vi "rhythm game.vi"() -> ()   [LabVIEW 2023]
uses:
  <vilib>/numeric/Random Number (Range) DBL.vi
  be73d2ca-6044-4015-8fdc-046309639c3a.vi
  e82d1244-044b-4f16-bbdc-f3884a827bcd.vi
  <vilib>/Utility/inputDevices.llb/keyboardAcquire.vi
panel:
  out "fg":picture
  in  "stop":bool
  out "bg":picture
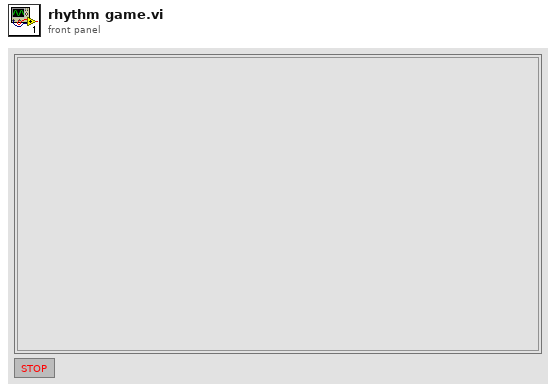
[diagram p1: front panel]
types:
  T1 = cluster{"1st rail":cluster{"key":enum16{"0", "1", "2", "3", "4", "5", "6", "7", "8", "9", "A", "B", "C", "D", "E", "F", "G", "H", "I", "J", "K", "L", "M", "N", "O", "P", "Q", "R", "S", "T", "U", "V", "W", "X", "Y", "Z", "F1", "F2", "F3", "F4", "F5", "F6", "F7", "F8", "F9", "F10", "F11", "F12", "F13", "F14", "F15", "ADD", "BACK", "BACKSLASH", "CAPITAL", "COMMA", "DECIMAL", "DELETE", "DIVIDE", "DOWN", "END", "EQUALS", "ESCAPE", "GRAVE (`)", "HOME", "INSERT", "LBRACKET", "LCONTROL", "LEFT", "L ALT", "LSHIFT", "LWIN", "MINUS", "MULTIPLY", "NEXT", "NUMLOCK", "NUMPAD_0", "NUMPAD_1", "NUMPAD_2", "NUMPAD_3", "NUMPAD_4", "NUMPAD_5", "NUMPAD_6", "NUMPAD_7", "NUMPAD_8", "NUMPAD_9", "PAUSE", "PERIOD", "PRIOR (PG UP)", "RBRACKET", "RCONTROL", "RETURN", "RIGHT", "R ALT", "RSHIFT", "RWIN", "SCROLL", "SEMICOLON", "SLASH", "SPACE", "SUBTRACT", "TAB", "UP", "ENTER (num pad)", "' (quote)"}, "note index":i32, "note acc":i32}, "2nd rail":cluster{"key":enum16{"0", "1", "2", "3", "4", "5", "6", "7", "8", "9", "A", "B", "C", "D", "E", "F", "G", "H", "I", "J", "K", "L", "M", "N", "O", "P", "Q", "R", "S", "T", "U", "V", "W", "X", "Y", "Z", "F1", "F2", "F3", "F4", "F5", "F6", "F7", "F8", "F9", "F10", "F11", "F12", "F13", "F14", "F15", "ADD", "BACK", "BACKSLASH", "CAPITAL", "COMMA", "DECIMAL", "DELETE", "DIVIDE", "DOWN", "END", "EQUALS", "ESCAPE", "GRAVE (`)", "HOME", "INSERT", "LBRACKET", "LCONTROL", "LEFT", "L ALT", "LSHIFT", "LWIN", "MINUS", "MULTIPLY", "NEXT", "NUMLOCK", "NUMPAD_0", "NUMPAD_1", "NUMPAD_2", "NUMPAD_3", "NUMPAD_4", "NUMPAD_5", "NUMPAD_6", "NUMPAD_7", "NUMPAD_8", "NUMPAD_9", "PAUSE", "PERIOD", "PRIOR (PG UP)", "RBRACKET", "RCONTROL", "RETURN", "RIGHT", "R ALT", "RSHIFT", "RWIN", "SCROLL", "SEMICOLON", "SLASH", "SPACE", "SUBTRACT", "TAB", "UP", "ENTER (num pad)", "' (quote)"}, "note index":i32, "note acc":i32}}
  T2 = cluster{"song name":string, "bpm":i32, "duration":i32, "1st rail":cluster{"note type":string, "position":dbl}[], "2nd rail":cluster{"note type":string, "position":dbl}[], "scrolling speed":dbl}
  T3 = enum16{"song select", "difficulty select", "gameplay", "result"}
  T4 = enum16{"0", "1", "2", "3", "4", "5", "6", "7", "8", "9", "A", "B", "C", "D", "E", "F", "G", "H", "I", "J", "K", "L", "M", "N", "O", "P", "Q", "R", "S", "T", "U", "V", "W", "X", "Y", "Z", "F1", "F2", "F3", "F4", "F5", "F6", "F7", "F8", "F9", "F10", "F11", "F12", "F13", "F14", "F15", "ADD", "BACK", "BACKSLASH", "CAPITAL", "COMMA", "DECIMAL", "DELETE", "DIVIDE", "DOWN", "END", "EQUALS", "ESCAPE", "GRAVE (`)", "HOME", "INSERT", "LBRACKET", "LCONTROL", "LEFT", "L ALT", "LSHIFT", "LWIN", "MINUS", "MULTIPLY", "NEXT", "NUMLOCK", "NUMPAD_0", "NUMPAD_1", "NUMPAD_2", "NUMPAD_3", "NUMPAD_4", "NUMPAD_5", "NUMPAD_6", "NUMPAD_7", "NUMPAD_8", "NUMPAD_9", "PAUSE", "PERIOD", "PRIOR (PG UP)", "RBRACKET", "RCONTROL", "RETURN", "RIGHT", "R ALT", "RSHIFT", "RWIN", "SCROLL", "SEMICOLON", "SLASH", "SPACE", "SUBTRACT", "TAB", "UP", "ENTER (num pad)", "' (quote)"}[]
  T5 = cluster{"combo":i32, "max combo":i32, "note acc":i32[], dbl}
  T6 = cluster{"combo":i32, "max combo":i32, "note acc":i32[], "progress":dbl}
  T7 = cluster{dbl, "note acc":cluster{i32, i32}, "new next note":cluster{"1st rail":i32, "2nd rail":i32}, "combo":i32, "score":i32}
  T8 = cluster{enum16{"0", "1"}, enum16{"easy", "hard"}}
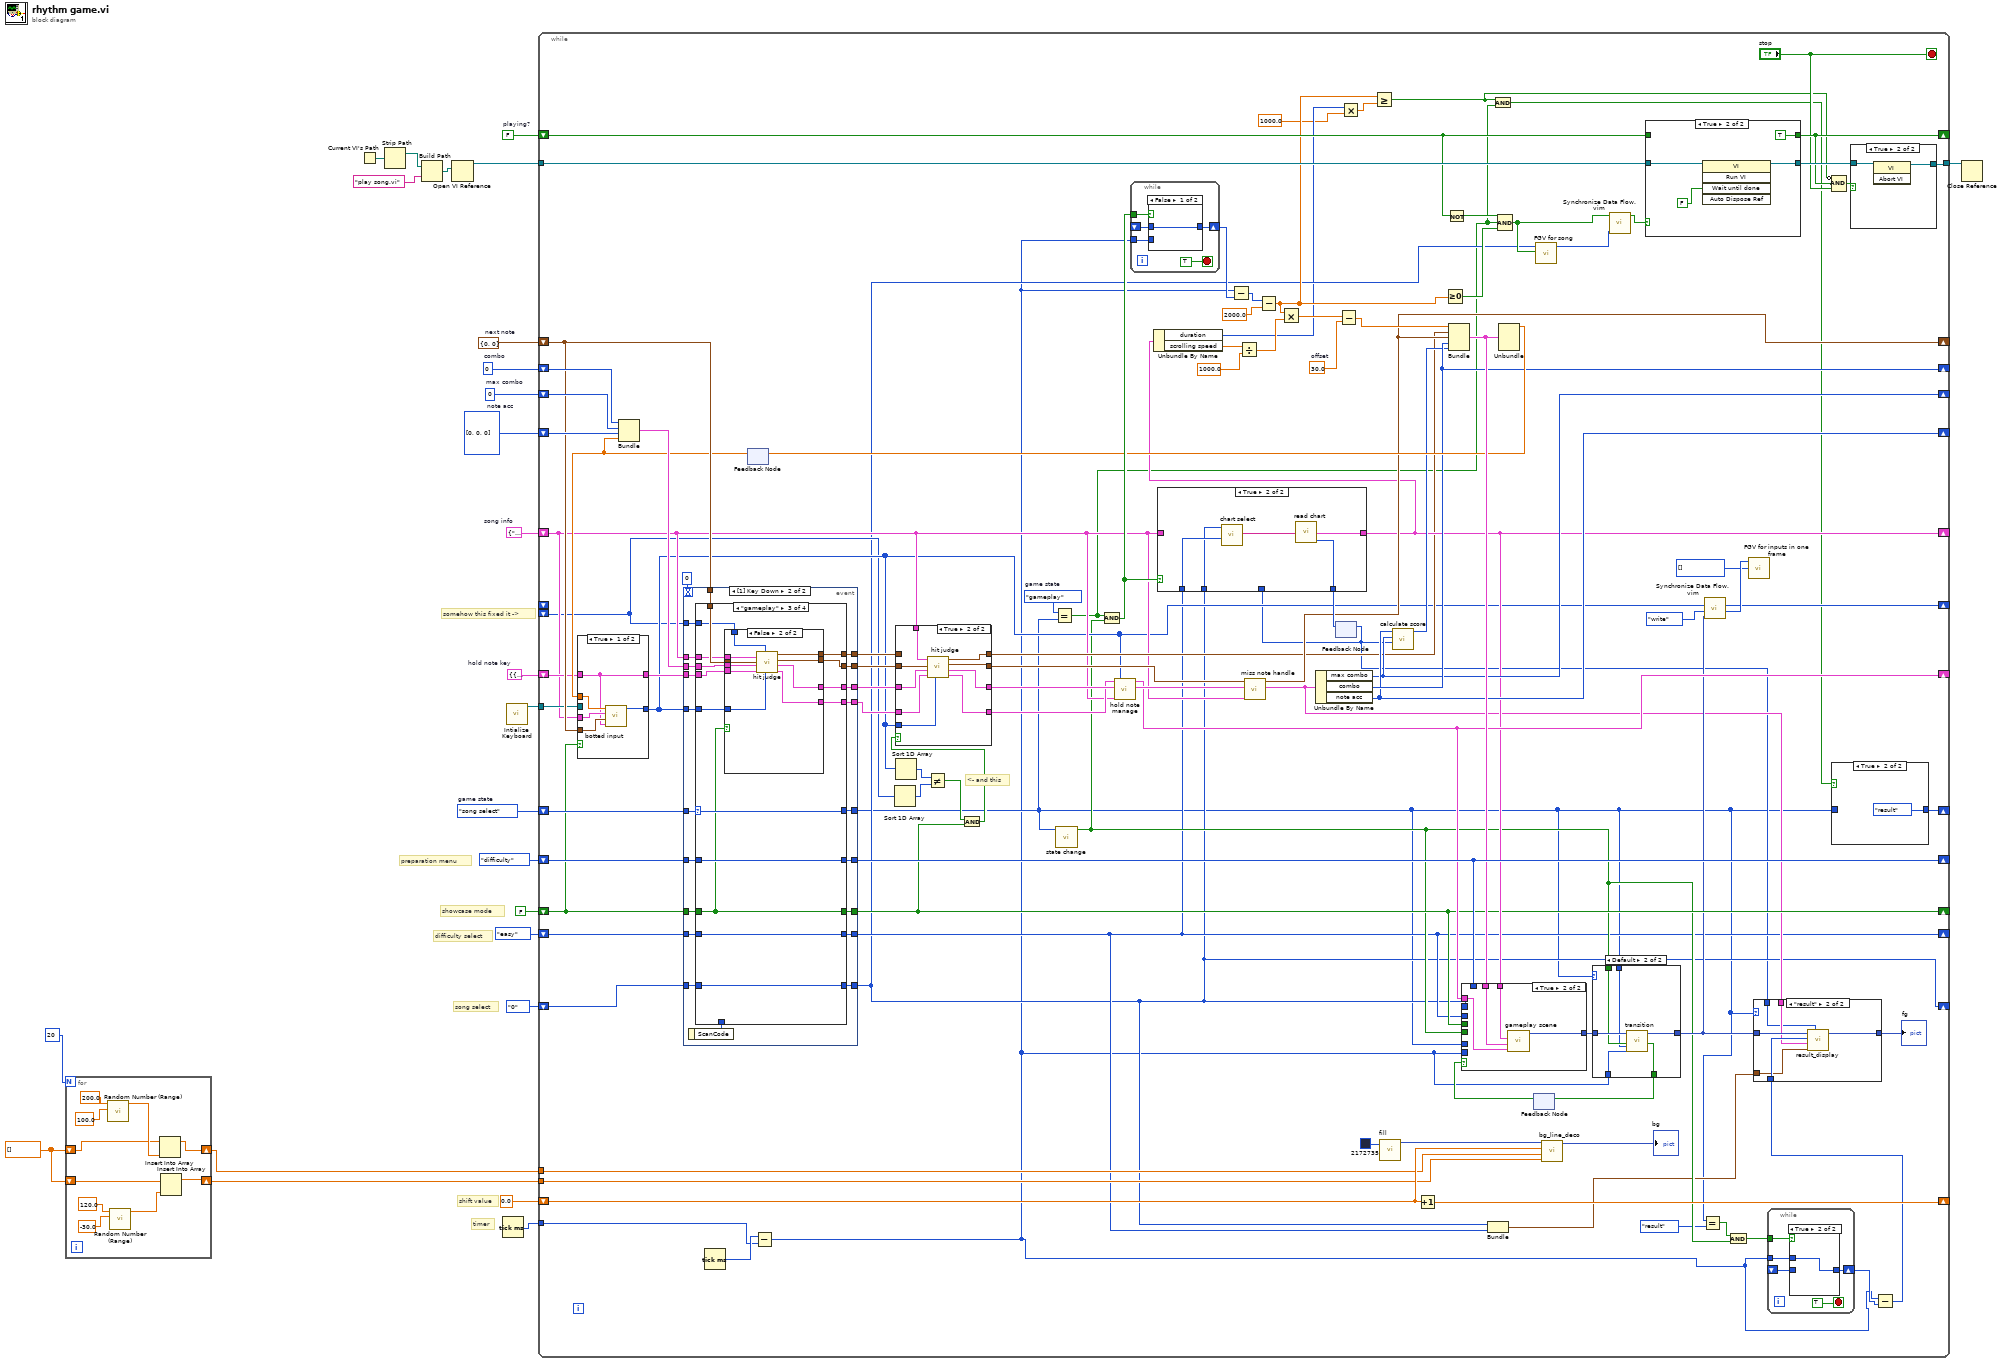
[diagram p0: block diagram]
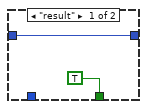
[diagram p2: hidden frame]
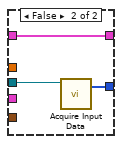
[diagram p8: hidden frame]
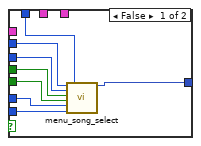
[diagram p9: hidden frame]
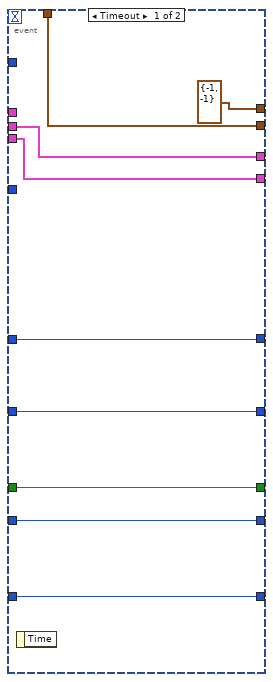
[diagram p13: hidden frame]
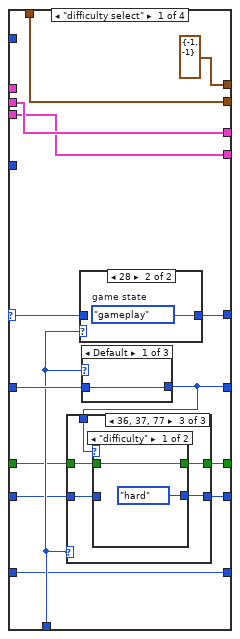
[diagram p14: hidden frame]
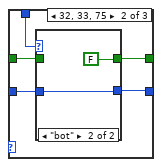
[diagram p16: hidden frame]
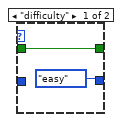
[diagram p17: hidden frame]
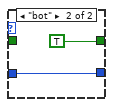
[diagram p18: hidden frame]
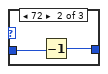
[diagram p20: hidden frame]
diagram:
  w2 = T1 {"1st rail"={"key"=enum."0", "note index"=-1, "note acc"=-1}, "2nd rail"={"key"=enum."0", "note index"=-1, "note acc"=-1}}  # hold note key
  w3 = 0  # max combo
  w4 = i32[] [0, 0, 0]  # note acc
  w5 = cluster{"1st rail":i32, "2nd rail":i32} {"1st rail"=0, "2nd rail"=0}  # next note
  w6 = T2 {"song name"="", "bpm"=0, "duration"=0, "1st rail"=[], "2nd rail"=[], "scrolling speed"=0.0}  # song info
  w7 = 0  # combo
  w9 = FALSE  # playing?
  w19 = T3."song select"  # game state
  w23 = dbl[] []
  # "somehow this fixed it ->"
  # "preparation menu"
  # "showcase mode"
  # "difficulty select"
  # "timer"
  # "song select"
  # "shift value"
  n1 = for {
    N: 20 -> [_]
    shift-right: [w31] -> w22
    shift-left: w23 -> [w32]
    shift-right: [w26] -> w21
    shift-left: w23 -> [w28]
    n2 = call-poly <vilib>:"Random Number (Range).vi"("lower bound (0)"=100.0, "upper bound (100)"=200.0) -> ("number"=w33:dbl)  [unwired: 9 in]
    n3 = call-poly <vilib>:"Random Number (Range).vi"("lower bound (0)"=-30.0, "upper bound (100)"=120.0) -> ("number"=w27:dbl)  [unwired: 9 in]
    n4 = Insert Into Array(array=w32, new element=w33) -> (w31:dbl[])  [unwired: 1 in]
    n5 = Insert Into Array(array=w28, new element=w27) -> (w26:dbl[])  [unwired: 1 in]
  }
  n6 = Current VI's Path() -> (path=w14:path)
  n7 = Strip Path(path=w14) -> (stripped path=w13:path)  [unwired: 1 out]
  n8 = Build Path(base path=w13, name or relative path="play song.vi") -> (appended path=w11:path)
  n9 = Open VI Reference(vi path=w11) -> (vi reference=w10:refnum<vi>)  [unwired: 5 in, 1 out]
  n10 = Tick Count (ms)() -> (millisecond timer value=w18:u32)
  n11 = call <vilib>:"Intialize Keyboard.vi"() -> ("device ID"=w1:refnum<k1>)  [unwired: 10 in, 1 out]
  n12 = while {
    shift-right: [w131] -> _
    shift-left: 0.0 -> [w138]
    tunnel: w22 -> [w137]
    tunnel: w21 -> [w136]
    shift-right: [w47] -> _
    shift-left: enum16{"0", "1"}."0" -> [w134]
    shift-right: [w57] -> _
    shift-left: w19 -> [w132]
    tunnel: w18 -> [w129]
    shift-right: [w48] -> _
    shift-left: enum16{"easy", "hard"}."easy" -> [w128]
    shift-right: [w68] -> _
    shift-left: FALSE -> [w91]
    shift-right: [w114] -> _
    shift-left: enum16{"difficulty", "bot"}."difficulty" -> [w127]
    tunnel: w10 -> [w122]
    shift-right: [w70] -> _
    shift-left: w9 -> [w121]
    shift-right: [w97] -> _
    shift-left: w5 -> [w90]
    tunnel: [w72] -> w8
    shift-right: [w95] -> _
    shift-left: w6 -> [w77]
    shift-right: [w108] -> _
    shift-left: w7 -> [w104]
    shift-right: [w107] -> _
    shift-left: w4 -> [w112]
    shift-right: [w96] -> _
    shift-left: w2 -> [w87]
    shift-right: [w102] -> _
    shift-left: w3 -> [w103]
    tunnel: w1 -> [w88]
    shift-right: [w69] -> _
    shift-left: _ -> [_]
    shift-left: _ -> [w62]
    stop <- "stop" stop-if-true
    w92 = T4 [] items=["0", "1", "2", "3", "4", "5", "6", "7", "8", "9", "A", "B", "C", "D", "E", "F", "G", "H", "I", "J", "K", "L", "M", "N", "O", "P", "Q", "R", "S", "T", "U", "V", "W", "X", "Y", "Z", "F1", "F2", "F3", "F4", "F5", "F6", "F7", "F8", "F9", "F10", "F11", "F12", "F13", "F14", "F15", "ADD", "BACK", "BACKSLASH", "CAPITAL", "COMMA", "DECIMAL", "DELETE", "DIVIDE", "DOWN", "END", "EQUALS", "ESCAPE", "GRAVE (`)", "HOME", "INSERT", "LBRACKET", "LCONTROL", "LEFT", "L ALT", "LSHIFT", "LWIN", "MINUS", "MULTIPLY", "NEXT", "NUMLOCK", "NUMPAD_0", "NUMPAD_1", "NUMPAD_2", "NUMPAD_3", "NUMPAD_4", "NUMPAD_5", "NUMPAD_6", "NUMPAD_7", "NUMPAD_8", "NUMPAD_9", "PAUSE", "PERIOD", "PRIOR (PG UP)", "RBRACKET", "RCONTROL", "RETURN", "RIGHT", "R ALT", "RSHIFT", "RWIN", "SCROLL", "SEMICOLON", "SLASH", "SPACE", "SUBTRACT", "TAB", "UP", "ENTER (num pad)", "' (quote)"] ("read out inputs")
    w99 = 30.0  # offset
    w126 = T3."gameplay"  # game state
    # "<- and this"
    n13 = Tick Count (ms)() -> (millisecond timer value=w130:u32)
    n14 = feedback #1() -> (w89:dbl)  [unwired: 1 in]
    n15 = case shown="True" w91 {
      tunnel: [w182 w188] -> w65
      tunnel: w77 -> [w184 _]
      tunnel: w90 -> [w183 _]
      tunnel: w89 -> [w185 _]
      tunnel: w88 -> [_ w187]
      tunnel: w87 -> [w181 w186]
      tunnel: [w181 w186] -> w86
      frame True {
        n16 = call "botted input.vi"("hold note key"=w181, "next note"=w183, "song info"=w184, "progress"=w185) -> ("keys pressed"=w182:T4)  [unwired: 7 in]
      }
      frame False {
        n17 = call-poly <vilib>:"Acquire Input Data.vi"("device ID"=w187) -> ("keys pressed"=w188:T4)  [unwired: 16 in, 2 out]
      }
    }
    n18 = Bundle("combo"=w104, "max combo"=w103, "note acc"=w112, w89) -> (w111:T5)  [unwired: 1 in]
    n19 = event shown="[1] Key Down" {
      selector: _ -> [_ _]
      dyn-events: _ -> [_ _]
      timeout: 0 -> [_ _]
      tunnel: w134 -> [w229 w250]
      tunnel: [w229 w249] -> w47
      tunnel: w132 -> [w228 w247]
      tunnel: [w228 w246] -> w44
      tunnel: w128 -> [w225 w241]
      tunnel: w91 -> [w226 w243]
      tunnel: w127 -> [w227 w245]
      tunnel: [w227 w244] -> w114
      tunnel: [w226 w242] -> w68
      tunnel: [w225 w240] -> w48
      tunnel: w90 -> [w224 w239]
      tunnel: w77 -> [_ w238]
      tunnel: w111 -> [w222 w237]
      tunnel: w65 -> [_ w236]
      tunnel: [cluster{i32, i32} {-1, -1} ("note acc") w235] -> w85
      tunnel: [w224 w234] -> w83
      tunnel: [w222 w233] -> w81
      tunnel: [w221 w232] -> w79
      tunnel: w86 -> [w221 w231]
      tunnel: w62 -> [_ w230]
      event Timeout {
        n20 = event-data() -> ()  [unwired: 1 in, 1 out]
      }
      event Key Down {
        n21 = event-data() -> ("ScanCode"=w248:i16)  [unwired: 1 in]
        n22 = case shown="\"gameplay\"" w247 {
          selector: w247 -> [w263 w300 w324 w347]
          tunnel: w250 -> [w255 w303 w325 w348]
          tunnel: [w255 w302 w325 w348] -> w249
          tunnel: w248 -> [w261 w301 _ _]
          tunnel: [w262 w299 w324 w347] -> w246
          tunnel: w245 -> [w264 w298 w323 w346]
          tunnel: [w256 w298 w323 w346] -> w244
          tunnel: w243 -> [w260 w297 w312 w345]
          tunnel: [w259 w297 w312 w345] -> w242
          tunnel: w241 -> [w258 w296 w322 w344]
          tunnel: [w257 w296 w322 w344] -> w240
          tunnel: w239 -> [w254 w295 w321 w343]
          tunnel: w238 -> [_ _ w320 _]
          tunnel: w237 -> [w252 w293 w319 w341]
          tunnel: w236 -> [_ _ w318 _]
          tunnel: [cluster{i32, i32} {-1, -1} ("note acc") cluster{i32, i32} {-1, -1} ("note acc") w317 cluster{i32, i32} {-1, -1} ("note acc")] -> w235
          tunnel: [w254 w295 w316 w343] -> w234
          tunnel: [w252 w293 w315 w341] -> w233
          tunnel: [w251 w292 w314 w340] -> w232
          tunnel: w231 -> [w251 w292 w313 w340]
          tunnel: w230 -> [_ _ w311 _]
          frame "difficulty select" {
            n23 = case shown="28" w261 {
              tunnel: w263 -> [w285 _]
              tunnel: [w285 w286] -> w262
              frame Default {
              }
              frame 28 {
                w286 = T3."gameplay"  # game state
              }
            }
            n24 = case shown="Default" w261 {
              tunnel: w264 -> [w287 w289 w291]
              tunnel: [w287 w288 w290] -> w256
              frame Default {
              }
              frame 72 {
                n25 = Decrement(x=w289) -> (x-1=w288:enum16{"difficulty", "bot"})
              }
              frame 80 {
                n26 = Increment(x=w291) -> (x+1=w290:enum16{"difficulty", "bot"})
              }
            }
            n27 = case shown="36, 37, 77" w261 {
              tunnel: w260 -> [w266 w269 w278]
              tunnel: [w266 w268 w277] -> w259
              tunnel: w258 -> [w265 w267 w276]
              tunnel: [w265 w271 w280] -> w257
              tunnel: w256 -> [_ w270 w279]
              frame Default {
              }
              frame 32, 33, 75 {
                n28 = case shown="\"bot\"" w270 {
                  tunnel: [enum16{"easy", "hard"}."easy" w275] -> w271
                  tunnel: w269 -> [w272 _]
                  tunnel: [w272 FALSE] -> w268
                  tunnel: w267 -> [_ w275]
                  frame "difficulty" {
                  }
                  frame "bot" {
                  }
                }
              }
              frame 36, 37, 77 {
                n29 = case shown="\"difficulty\"" w279 {
                  tunnel: [enum16{"easy", "hard"}."hard" w283] -> w280
                  tunnel: w278 -> [w282 _]
                  tunnel: [w282 TRUE] -> w277
                  tunnel: w276 -> [_ w283]
                  frame "difficulty" {
                  }
                  frame "bot" {
                  }
                }
              }
            }
          }
          frame "song select" {
            n30 = case shown="28" w301 {
              tunnel: w300 -> [w304 _]
              tunnel: [w304 w305] -> w299
              frame 0, Default {
              }
              frame 28 {
                w305 = T3."difficulty select"  # game state
              }
            }
            n31 = case shown="36, 37, 77" w301 {
              tunnel: w303 -> [w306 w308 w309]
              tunnel: [w307 w308 w310] -> w302
              frame 32, 33, 75 {
                n32 = Decrement(x=w306) -> (x-1=w307:enum16{"0", "1"})
              }
              frame Default {
              }
              frame 36, 37, 77 {
                n33 = Increment(x=w309) -> (x+1=w310:enum16{"0", "1"})
              }
            }
          }
          frame "gameplay" {
            n34 = case shown="False" w312 {
              tunnel: w321 -> [w327 w339]
              tunnel: w320 -> [_ w338]
              tunnel: w319 -> [w328 w337]
              tunnel: w318 -> [_ w336]
              tunnel: [cluster{i32, i32} {-1, -1} ("note acc") w335] -> w317
              tunnel: [w327 w334] -> w316
              tunnel: [w328 w333] -> w315
              tunnel: [w329 w332] -> w314
              tunnel: w313 -> [w329 w331]
              tunnel: w311 -> [_ w330]
              frame True {
              }
              frame False {
                n35 = call "hit judge.vi"("keys pressed"=w336, "click last frame"=w330, "hold note key"=w331, "score info"=w337, "next note"=w339, "song info"=w338) -> ("hold note key"=w332:T1, "new score info"=w333:T6, "next note"=w334:cluster{"1st rail":i32, "2nd rail":i32}, "note acc"=w335:cluster{i32, i32})  [unwired: 2 in]
              }
            }
          }
          frame "result" {
          }
        }
      }
    }
    n36 = Subtract(x=w130, y=w129) -> (x-y=w38:u32)
    n37 = Sort 1D Array(array=w62) -> (sorted array=w64:T4)
    n38 = Sort 1D Array(array=w65) -> (sorted array=w63:T4)
    n39 = Not Equal?(x=w63, y=w64) -> (x != y?=w67:bool)
    n40 = And(x=w67, y=w68) -> (x .and. y?=w66:bool)
    n41 = case shown="True" w66 {
      tunnel: [w171 w177] -> w84
      tunnel: w85 -> [w171 _]
      tunnel: [w170 w178] -> w82
      tunnel: w83 -> [w170 w174]
      tunnel: [w169 w176] -> w80
      tunnel: w81 -> [w169 w172]
      tunnel: [w168 w175] -> w78
      tunnel: w79 -> [w168 w173]
      tunnel: w65 -> [_ w180]
      tunnel: w77 -> [_ w179]
      frame False {
      }
      frame True {
        n42 = call "hit judge.vi"("keys pressed"=w180, "hold note key"=w173, "score info"=w172, "next note"=w174, "song info"=w179) -> ("hold note key"=w175:T1, "new score info"=w176:T6, "next note"=w178:cluster{"1st rail":i32, "2nd rail":i32}, "note acc"=w177:cluster{i32, i32})  [unwired: 3 in]
      }
    }
    n43 = Equal?(x=w126, y=w44) -> (x = y?=w40:bool)
    n44 = call "state change.vi"("game state"=w44) -> ("T/F"=w54:bool)  [unwired: 10 in]
    n45 = And(x=w40, y=w54) -> (x .and. y?=w125:bool)
    n46 = call "hold note manage.vi"("keys pressed"=w65, "song info"=w77, "score info"=w80, "hold note key"=w78) -> ("new score info"=w98:T6, "new hold note key"=w96:T1)  [unwired: 6 in]
    n47 = while {
      tunnel: w38 -> [w209]
      tunnel: w125 -> [w210]
      shift-right: [w208] -> w61
      shift-left: _ -> [w207]
      stop <- TRUE stop-if-true
      n48 = case shown="False" w210 {
        tunnel: w209 -> [_ w213]
        tunnel: [w212 w213] -> w208
        tunnel: w207 -> [w212 _]
        frame False {
        }
        frame True {
        }
      }
    }
    n49 = Subtract(x=w38, y=w61) -> (x-y=w124:u32)
    n50 = call "miss note handle.vi"("song info"=w77, "score info"=w98, "next note"=w82) -> ("new score info"=w49:T6, "new next note"=w97:cluster{"1st rail":i32, "2nd rail":i32})  [unwired: 7 in]
    n51 = Subtract(x=w124, y=2000.0) -> (x-y=w60:dbl)
    n52 = Unbundle By Name(w49) -> ("max combo"=w102:i32, "combo"=w108:i32, "note acc"=w107:i32[])
    n53 = feedback #2() -> (w45:i32)  [unwired: 1 in]
    n54 = case shown="True" w125 {
      tunnel: [w215 w220] -> w95
      tunnel: w77 -> [w215 _]
      tunnel: [w214 w219] -> w105
      tunnel: w45 -> [w214 _]
      tunnel: w48 -> [_ w217]
      tunnel: w47 -> [_ w216]
      frame False {
      }
      frame True {
        n55 = call "chart select.vi"("difficulty"=w217, "song"=w216) -> ("file name"=w218:string)  [unwired: 9 in]
        n56 = call "read chart.vi"("file name (.txt)"=w218) -> ("note count"=w219:i32, "song info"=w220:T2)  [unwired: 3 in]
      }
    }
    n57 = Unbundle By Name(w95) -> ("duration"=w42:i32, "scrolling speed"=w113:dbl)
    n58 = Divide(x=w113, y=1000.0) -> (x/y=w118:dbl)
    n59 = Multiply(x=w60, y=w118) -> (x*y=w101:dbl)
    n60 = feedback-in #2(w105) -> ()
    n61 = Subtract(x=w101, y=w99) -> (x-y=w100:dbl)
    n62 = Multiply(x=w42, y=1000.0) -> (x*y=w43:dbl)
    n63 = Greater Or Equal?(x=w60, y=w43) -> (x >= y?=w37:bool)
    n64 = call "fill.vi"("color (black)"=u32 2172735 ("color(black)")) -> ("new picture"=w139:picture)  [unwired: 10 in]
    n65 = call "calculate score.vi"("note count"=w45, "max combo"=w102, "note acc"=w107) -> ("score"=w106:i32)  [unwired: 7 in, 1 out]
    n66 = Increment(x=w138) -> (x+1=w131:dbl)
    n67 = Greater Or Equal To 0?(x=w60) -> (x >= 0?=w120:bool)
    n68 = Not(x=w121) -> (.not. x?=w59:bool)
    n69 = Bundle(w100, "note acc"=w84, "new next note"=w97, "combo"=w108, "score"=w106) -> (w110:T7)  [unwired: 1 in]
    n70 = Bundle(w47, w48) -> (w46:T8)  [unwired: 1 in]
    n71 = Compound Arithmetic op=AND(w37, w40) -> (w56:bool)
    n72 = Compound Arithmetic op=AND(w59, w40, w120) -> (w76:bool)
    n73 = Unbundle(w110) -> (w109:dbl)  [unwired: 4 out]
    n74 = feedback-in #1(w109) -> ()
    n75 = feedback #3() -> (w115:bool)  [unwired: 1 in]
    n76 = case shown="True" w115 {
      tunnel: [w189 w200] -> w117
      tunnel: w95 -> [_ w199]
      tunnel: w110 -> [_ w198]
      tunnel: w47 -> [w196 _]
      tunnel: w48 -> [w195 _]
      tunnel: w68 -> [w194 _]
      tunnel: w54 -> [w193 _]
      tunnel: w44 -> [w192 _]
      tunnel: w38 -> [w191 _]
      tunnel: w114 -> [w190 _]
      tunnel: w96 -> [_ w197]
      frame False {
        n77 = call "menu_song_select.vi"("song id"=w196, "difficulty"=w195, "showcase"=w194, "state change"=w193, "game state"=w192, "timer"=w191, "prepare menu"=w190) -> ("new picture"=w189:picture)  [unwired: 11 in, 1 out]
      }
      frame True {
        n78 = call "gameplay scene.vi"("hold note key"=w197, "gameplay info"=w198, "chart info"=w199) -> ("new picture"=w200:picture)  [unwired: 8 in]
      }
    }
    n79 = call "FGV for song.vi"("mode"=w76, "write song"=w47) -> ("read song"=w74:enum16{"0", "1"})  [unwired: 9 in]
    n80 = call "bg_line_deco.vi"("line slope"=w136, "line pos"=w137, "shift value"=w138, "new picture in"=w139) -> ("new picture out"=→"bg":picture)  [unwired: 7 in]
    n81 = case shown="Default" w44 {
      tunnel: w117 -> [w142 w148]
      tunnel: [TRUE w147] -> w116
      tunnel: [w142 w146] -> w55
      tunnel: w54 -> [_ w145]
      tunnel: w44 -> [_ w144]
      tunnel: w38 -> [_ w143]
      frame "result" {
      }
      frame Default {
        n82 = call "transition.vi"("new picture in"=w148, "state change"=w145, "game state"=w144, "timer"=w143) -> ("new picture out"=w146:picture, "change (of) scene"=w147:bool)  [unwired: 14 in]
      }
    }
    n83 = feedback-in #3(w116) -> ()
    n84 = call "Synchronize Data Flow.vim"("input 4"=w74, "input 1"=w76) -> ("output 1"=w75:bool)  [unwired: 2 in, 3 out]
    n85 = case shown="True" w75 {
      tunnel: w122 -> [w201 w203]
      tunnel: w121 -> [w202 _]
      tunnel: [w202 TRUE ("Wait Until Done")] -> w70
      tunnel: [w201 w204] -> w73
      frame False {
      }
      frame True {
        n86 = invoke class="VI" method="Run VI"(reference=w203, "Wait until done"=FALSE ("Wait Until Done")) -> (reference out=w204:refnum<vi>)  [unwired: 3 in, 4 out]
      }
    }
    n87 = Equal?(x=w44, y=T3."result") -> (x = y?=w53:bool)
    n88 = call "Synchronize Data Flow.vim"("input 4"=w55, "input 3"=enum16{"read", "write"}."write" ("mode"), "input 2"=w65) -> ("output 3"=w93:enum16{"read", "write"}, "output 2"=w69:T4)  [unwired: 1 in, 2 out]
    n89 = And(x=w53, y=w54) -> (x .and. y?=w51:bool)
    n90 = call "FGV for inputs in one frame.vi"("write in key"=w92, "mode"=w93) -> ()  [unwired: 9 in, 1 out]
    n91 = while {
      tunnel: w51 -> [w152]
      tunnel: w38 -> [w151]
      shift-right: [w150] -> w39
      shift-left: _ -> [w149]
      stop <- TRUE stop-if-true
      n92 = case shown="True" w152 {
        tunnel: w151 -> [_ w155]
        tunnel: [w154 w155] -> w150
        tunnel: w149 -> [w154 _]
        frame False {
        }
        frame True {
        }
      }
    }
    n93 = Compound Arithmetic op=AND(invert w37, w70, "stop") -> (w71:bool)
    n94 = case shown="True" w56 {
      tunnel: w44 -> [w163 _]
      tunnel: [w163 T3."result" ("game state")] -> w57
      frame False {
      }
      frame True {
      }
    }
    n95 = case shown="True" w71 {
      tunnel: w73 -> [w165 w167]
      tunnel: [w165 w166] -> w72
      frame False {
      }
      frame True {
        n96 = invoke class="VI" method="Abort VI"(reference=w167) -> (reference out=w166:refnum<vi>)  [unwired: 2 in, 2 out]
      }
    }
    n97 = Subtract(x=w38, y=w39) -> (x-y=w50:u32)
    n98 = case shown="\"result\"" w44 {
      tunnel: w55 -> [w156 w162]
      tunnel: [w156 w161] -> w36
      tunnel: w50 -> [_ w160]
      tunnel: w49 -> [_ w159]
      tunnel: w46 -> [_ w158]
      tunnel: w45 -> [_ w157]
      frame Default {
      }
      frame "result" {
        n99 = call "result_display.vi"("note count"=w157, "lvl info"=w158, "score info"=w159, "timer"=w160, "new picture in"=w162) -> ("new picture"=w161:picture)  [unwired: 6 in]
      }
    }
    "fg" <- w36
  }
  n100 = Close Reference(reference=w8) -> ()  [unwired: 1 in, 1 out]
